vi "Show Window Change Detector.vi"(8 "error in (no error)":errorcluster, 10 "Show Window":bool, 11 "Progress Bar in":refnum<class "Progress Bar.lvclass">) -> (0 "error out":errorcluster, 2 "Changed?":bool, 3 "Progress Bar out":refnum<class "Progress Bar.lvclass">)   [LabVIEW 2020, in "Progress Bar.lvclass"]
doc: "Checks to see if the show window flag has changed\n\nCopyright: MGI\nAuthored by: Derek Trepanier"
uses:
  <userlib>/_MGI/User Interface/Progress Bar/Progress Bar.lvclass
  <userlib>/_MGI/User Interface/Progress Bar/Progress Bar.lvclass/Progress Bar.ctl
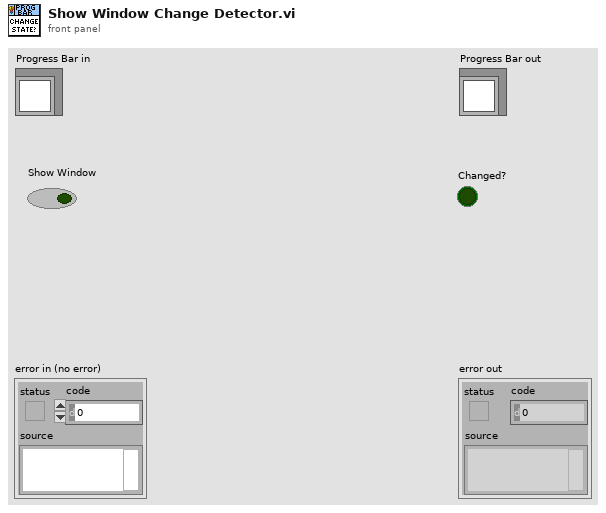
[diagram p1: front panel]
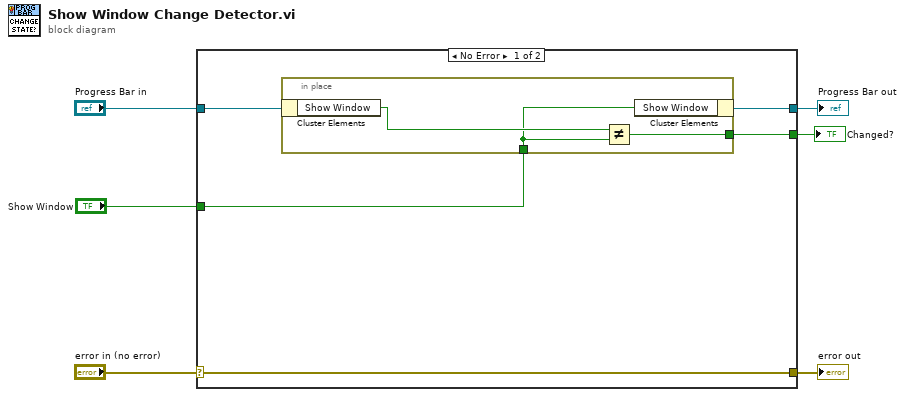
[diagram p0: block diagram]
diagram:
  n1 = case shown="No Error" "error in (no error)" {
    selector: "error in (no error)" -> [w11 w16]
    tunnel: [w11 w16] -> w5
    tunnel: [w7 w15] -> w3
    tunnel: "Progress Bar in" -> [w10 w15]
    tunnel: "Show Window" -> [w9 _]
    tunnel: [w8 _] -> w1
    frame No Error {
      n2 = in-place {
        in-place-border: w9 -> [w13]
        in-place-border: [w12] -> w8
        n3 = in-place-cluster #1(w10) -> ("Show Window"=w14:bool)
        n4 = Not Equal?(x=w14, y=w13) -> (x != y?=w12:bool)
        n5 = in-place-cluster #1("Show Window"=w13) -> (w7:refnum<class "Progress Bar.lvclass">)
      }
    }
    frame Error {
    }
  }
  "error out" <- w5
  "Progress Bar out" <- w3
  "Changed?" <- w1
